vi "Serialize.vi"(8 "error in (no error)":errorcluster, 11 "GObjectConverterBase in":refnum<class "GObjectConverterBase.lvclass">) -> (0 "error out":errorcluster, 2 "JSON":string, 3 "GObjectConverterBase out":refnum<class "GObjectConverterBase.lvclass">)   [LabVIEW 2017, in "GObjectConverterBase.lvclass"]
uses:
  GObjectConverterBase.lvclass
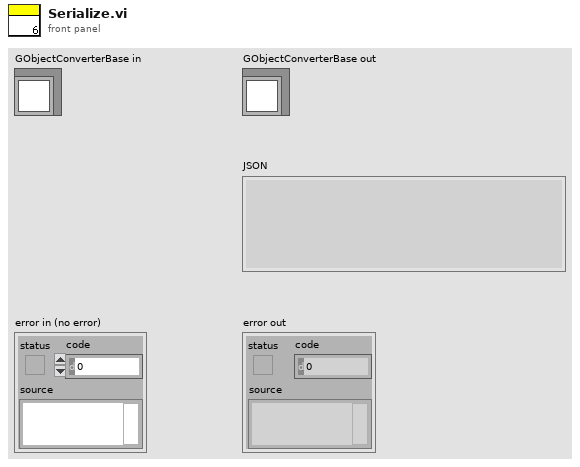
[diagram p1: front panel]
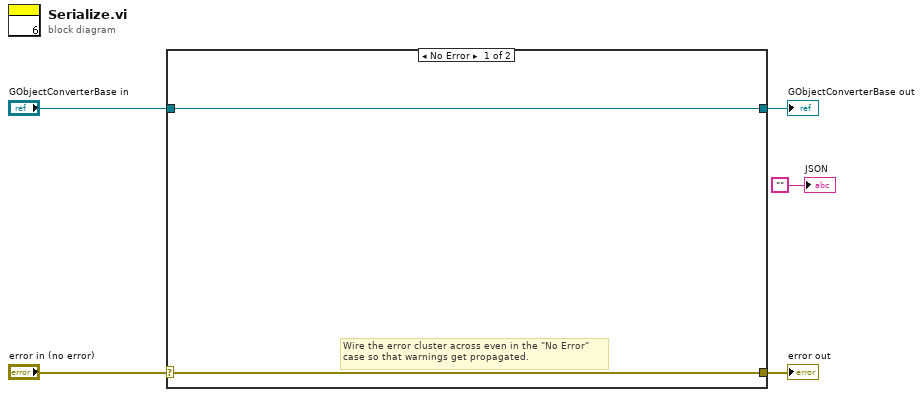
[diagram p0: block diagram]
diagram:
  n1 = case shown="No Error" "error in (no error)" {
    selector: "error in (no error)" -> [w6 w9]
    tunnel: [w6 w9] -> w4
    tunnel: [w7 w8] -> w2
    tunnel: "GObjectConverterBase in" -> [w7 w8]
    frame No Error {
      # "Wire the error cluster across even in the \"No Error\"\ncase so that warnings get propagated."
    }
    frame Error {
    }
  }
  "error out" <- w4
  "GObjectConverterBase out" <- w2
  "JSON" <- ""
